vi "Initialize TCS.vi"(8 "error in (no error)":errorcluster, 11 "AutoExp in":refnum<class "AutoExp.lvclass">) -> (0 "error out":errorcluster, 3 "AutoExp out":refnum<class "AutoExp.lvclass">)   [LabVIEW 2018, in "AutoExp.lvclass"]
uses:
  AutoExp.lvclass
  AutoExp.lvclass/AutoExp.ctl
  TCS/TCS.lvclass
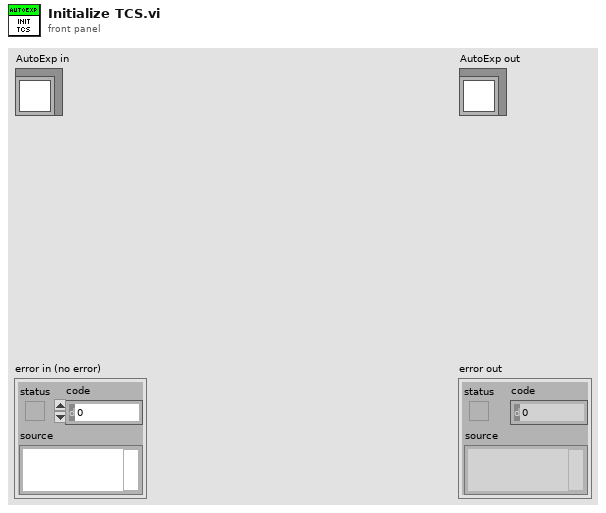
[diagram p1: front panel]
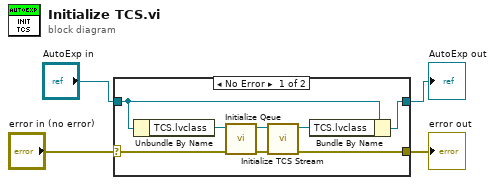
[diagram p0: block diagram]
diagram:
  n1 = case shown="No Error" "error in (no error)" {
    selector: "error in (no error)" -> [w12 w14]
    tunnel: [w11 w14] -> w3
    tunnel: [w7 w13] -> w1
    tunnel: "AutoExp in" -> [w6 w13]
    frame No Error {
      n2 = Unbundle By Name(w6) -> ("TCS.lvclass"=w8:refnum<class "TCS.lvclass">)
      n3 = call "Initialize Qeue.vi"("error in (no error)"=w12, "TCS in"=w8) -> ("error out"=w9:errorcluster, "TCS out"=w10:refnum<class "TCS.lvclass">)  [unwired: 8 in]
      n4 = call "Initialize TCS Stream.vi"("error in (no error)"=w9, "TCS in"=w10) -> ("error out"=w11:errorcluster, "TCS out"=w5:refnum<class "TCS.lvclass">)  [unwired: 8 in]
      n5 = Bundle By Name(cluster=w6, "TCS.lvclass"=w5) -> (w7:refnum<class "AutoExp.lvclass">)
    }
    frame Error {
    }
  }
  "error out" <- w3
  "AutoExp out" <- w1
